vi "App - analyze RUS V6.vi"() -> ()   [LabVIEW 2018] (continued)
Data\\Ultrasound\\LSCO\\LSCO22__130814c\\5_Cooling_2nd_try\\September_2014\\091714\\54.81600K_500_2500_2.10000V_0.00000T_Sep17-2014__10-18-21_001_091714.bin", "mod time(min)"=58230138.35, "file format"=enum."binary", "power(V)"=2.1, "Magn Field(T) "=0.0}, {"temperature"=54.752, "temperature str"="54.75200", "file path"=path "D:/Data/Ultrasound/LSCO/LSCO22__130814c/5_Cooling_2nd_try/September_2014/091714/54.75200K_500_2500_2.10000V_0.00000T_Sep17-2014__10-19-41_001_091714.bin", "last mod"=timestamp(3493808381 s since 1904-01-01), "file name str"="D:\\Data\\Ultrasound\\LSCO\\LSCO22__130814c\\5_Cooling_2nd_try\\September_2014\\091714\\54.75200K_500_2500_2.10000V_0.00000T_Sep17-2014__10-19-41_001_091714.bin", "mod time(min)"=58230139.68333333, "file format"=enum."binary", "power(V)"=2.1, "Magn Field(T) "=0.0}, {"temperature"=54.691, "temperature str"="54.69100", "file path"=path "D:/Data/Ultrasound/LSCO/LSCO22__130814c/5_Cooling_2nd_try/September_2014/091714/54.69100K_500_2500_2.10000V_0.00000T_Sep17-2014__10-21-00_001_091714.bin", "last mod"=timestamp(3493808460 s since 1904-01-01), "file name str"="D:\\Data\\Ultrasound\\LSCO\\LSCO22__130814c\\5_Cooling_2nd_try\\September_2014\\091714\\54.69100K_500_2500_2.10000V_0.00000T_Sep17-2014__10-21-00_001_091714.bin", "mod time(min)"=58230141.0, "file format"=enum."binary", "power(V)"=2.1, "Magn Field(T) "=0.0}, {"temperature"=54.628, "temperature str"="54.62800", "file path"=path "D:/Data/Ultrasound/LSCO/LSCO22__130814c/5_Cooling_2nd_try/September_2014/091714/54.62800K_500_2500_2.10000V_0.00000T_Sep17-2014__10-22-19_001_091714.bin", "last mod"=timestamp(3493808539 s since 1904-01-01), "file name str"="D:\\Data\\Ultrasound\\LSCO\\LSCO22__130814c\\5_Cooling_2nd_try\\September_2014\\091714\\54.62800K_500_2500_2.10000V_0.00000T_Sep17-2014__10-22-19_001_091714.bin", "mod time(min)"=58230142.31666667, "file format"=enum."binary", "power(V)"=2.1, "Magn Field(T) "=0.0}, {"temperature"=54.564, "temperature str"="54.56400", "file path"=path "D:/Data/Ultrasound/LSCO/LSCO22__130814c/5_Cooling_2nd_try/September_2014/091714/54.56400K_500_2500_2.10000V_0.00000T_Sep17-2014__10-23-39_001_091714.bin", "last mod"=timestamp(3493808619 s since 1904-01-01), "file name str"="D:\\Data\\Ultrasound\\LSCO\\LSCO22__130814c\\5_Cooling_2nd_try\\September_2014\\091714\\54.56400K_500_2500_2.10000V_0.00000T_Sep17-2014__10-23-39_001_091714.bin", "mod time(min)"=58230143.65, "file format"=enum."binary", "power(V)"=2.1, "Magn Field(T) "=0.0}, {"temperature"=54.505, "temperature str"="54.50500", "file path"=path "D:/Data/Ultrasound/LSCO/LSCO22__130814c/5_Cooling_2nd_try/September_2014/091714/54.50500K_500_2500_2.10000V_0.00000T_Sep17-2014__10-24-58_001_091714.bin", "last mod"=timestamp(3493808698 s since 1904-01-01), "file name str"="D:\\Data\\Ultrasound\\LSCO\\LSCO22__130814c\\5_Cooling_2nd_try\\September_2014\\091714\\54.50500K_500_2500_2.10000V_0.00000T_Sep17-2014__10-24-58_001_091714.bin", "mod time(min)"=58230144.96666667, "file format"=enum."binary", "power(V)"=2.1, "Magn Field(T) "=0.0}, {"temperature"=54.44, "temperature str"="54.44000", "file path"=path "D:/Data/Ultrasound/LSCO/LSCO22__130814c/5_Cooling_2nd_try/September_2014/091714/54.44000K_500_2500_2.10000V_0.00000T_Sep17-2014__10-26-18_001_091714.bin", "last mod"=timestamp(3493808778 s since 1904-01-01), "file name str"="D:\\Data\\Ultrasound\\LSCO\\LSCO22__130814c\\5_Cooling_2nd_try\\September_2014\\091714\\54.44000K_500_2500_2.10000V_0.00000T_Sep17-2014__10-26-18_001_091714.bin", "mod time(min)"=58230146.3, "file format"=enum."binary", "power(V)"=2.1, "Magn Field(T) "=0.0}, {"temperature"=54.375, "temperature str"="54.37500", "file path"=path "D:/Data/Ultrasound/LSCO/LSCO22__130814c/5_Cooling_2nd_try/September_2014/091714/54.37500K_500_2500_2.10000V_0.00000T_Sep17-2014__10-27-37_001_091714.bin", "last mod"=timestamp(3493808857 s since 1904-01-01), "file name str"="D:\\Data\\Ultrasound\\LSCO\\LSCO22__130814c\\5_Cooling_2nd_try\\September_2014\\091714\\54.37500K_500_2500_2.10000V_0.00000T_Sep17-2014__10-27-37_001_091714.bin", "mod time(min)"=58230147.61666667, "file format"=enum."binary", "power(V)"=2.1, "Magn Field(T) "=0.0}, {"temperature"=54.316, "temperature str"="54.31600", "file path"=path "D:/Data/Ultrasound/LSCO/LSCO22__130814c/5_Cooling_2nd_try/September_2014/091714/54.31600K_500_2500_2.10000V_0.00000T_Sep17-2014__10-28-56_001_091714.bin", "last mod"=timestamp(3493808936 s since 1904-01-01), "file name str"="D:\\Data\\Ultrasound\\LSCO\\LSCO22__130814c\\5_Cooling_2nd_try\\September_2014\\091714\\54.31600K_500_2500_2.10000V_0.00000T_Sep17-2014__10-28-56_001_091714.bin", "mod time(min)"=58230148.93333333, "file format"=enum."binary", "power(V)"=2.1, "Magn Field(T) "=0.0}, {"temperature"=54.252, "temperature str"="54.25200", "file path"=path "D:/Data/Ultrasound/LSCO/LSCO22__130814c/5_Cooling_2nd_try/September_2014/091714/54.25200K_500_2500_2.10000V_0.00000T_Sep17-2014__10-30-16_001_091714.bin", "last mod"=timestamp(3493809016 s since 1904-01-01), "file name str"="D:\\Data\\Ultrasound\\LSCO\\LSCO22__130814c\\5_Cooling_2nd_try\\September_2014\\091714\\54.25200K_500_2500_2.10000V_0.00000T_Sep17-2014__10-30-16_001_091714.bin", "mod time(min)"=58230150.266666666, "file format"=enum."binary", "power(V)"=2.1, "Magn Field(T) "=0.0}, {"temperature"=54.191, "temperature str"="54.19100", "file path"=path "D:/Data/Ultrasound/LSCO/LSCO22__130814c/5_Cooling_2nd_try/September_2014/091714/54.19100K_500_2500_2.10000V_0.00000T_Sep17-2014__10-31-35_001_091714.bin", "last mod"=timestamp(3493809095 s since 1904-01-01), "file name str"="D:\\Data\\Ultrasound\\LSCO\\LSCO22__130814c\\5_Cooling_2nd_try\\September_2014\\091714\\54.19100K_500_2500_2.10000V_0.00000T_Sep17-2014__10-31-35_001_091714.bin", "mod time(min)"=58230151.583333336, "file format"=enum."binary", "power(V)"=2.1, "Magn Field(T) "=0.0}, {"temperature"=54.128, "temperature str"="54.12800", "file path"=path "D:/Data/Ultrasound/LSCO/LSCO22__130814c/5_Cooling_2nd_try/September_2014/091714/54.12800K_500_2500_2.10000V_0.00000T_Sep17-2014__10-32-54_001_091714.bin", "last mod"=timestamp(3493809174 s since 1904-01-01), "file name str"="D:\\Data\\Ultrasound\\LSCO\\LSCO22__130814c\\5_Cooling_2nd_try\\September_2014\\091714\\54.12800K_500_2500_2.10000V_0.00000T_Sep17-2014__10-32-54_001_091714.bin", "mod time(min)"=58230152.9, "file format"=enum."binary", "power(V)"=2.1, "Magn Field(T) "=0.0}, {"temperature"=54.064, "temperature str"="54.06400", "file path"=path "D:/Data/Ultrasound/LSCO/LSCO22__130814c/5_Cooling_2nd_try/September_2014/091714/54.06400K_500_2500_2.10000V_0.00000T_Sep17-2014__10-34-14_001_091714.bin", "last mod"=timestamp(3493809254 s since 1904-01-01), "file name str"="D:\\Data\\Ultrasound\\LSCO\\LSCO22__130814c\\5_Cooling_2nd_try\\September_2014\\091714\\54.06400K_500_2500_2.10000V_0.00000T_Sep17-2014__10-34-14_001_091714.bin", "mod time(min)"=58230154.233333334, "file format"=enum."binary", "power(V)"=2.1, "Magn Field(T) "=0.0}, {"temperature"=54.004, "temperature str"="54.00400", "file path"=path "D:/Data/Ultrasound/LSCO/LSCO22__130814c/5_Cooling_2nd_try/September_2014/091714/54.00400K_500_2500_2.10000V_0.00000T_Sep17-2014__10-35-33_001_091714.bin", "last mod"=timestamp(3493809333 s since 1904-01-01), "file name str"="D:\\Data\\Ultrasound\\LSCO\\LSCO22__130814c\\5_Cooling_2nd_try\\September_2014\\091714\\54.00400K_500_2500_2.10000V_0.00000T_Sep17-2014__10-35-33_001_091714.bin", "mod time(min)"=58230155.55, "file format"=enum."binary", "power(V)"=2.1, "Magn Field(T) "=0.0}, {"temperature"=53.936, "temperature str"="53.93600", "file path"=path "D:/Data/Ultrasound/LSCO/LSCO22__130814c/5_Cooling_2nd_try/September_2014/091714/53.93600K_500_2500_2.10000V_0.00000T_Sep17-2014__10-36-53_001_091714.bin", "last mod"=timestamp(3493809413 s since 1904-01-01), "file name str"="D:\\Data\\Ultrasound\\LSCO\\LSCO22__130814c\\5_Cooling_2nd_try\\September_2014\\091714\\53.93600K_500_2500_2.10000V_0.00000T_Sep17-2014__10-36-53_001_091714.bin", "mod time(min)"=58230156.88333333, "file format"=enum."binary", "power(V)"=2.1, "Magn Field(T) "=0.0}, {"temperature"=53.874, "temperature str"="53.87400", "file path"=path "D:/Data/Ultrasound/LSCO/LSCO22__130814c/5_Cooling_2nd_try/September_2014/091714/53.87400K_500_2500_2.10000V_0.00000T_Sep17-2014__10-38-12_001_091714.bin", "last mod"=timestamp(3493809492 s since 1904-01-01), "file name str"="D:\\Data\\Ultrasound\\LSCO\\LSCO22__130814c\\5_Cooling_2nd_try\\September_2014\\091714\\53.87400K_500_2500_2.10000V_0.00000T_Sep17-2014__10-38-12_001_091714.bin", "mod time(min)"=58230158.2, "file format"=enum."binary", "power(V)"=2.1, "Magn Field(T) "=0.0}, {"temperature"=53.813, "temperature str"="53.81300", "file path"=path "D:/Data/Ultrasound/LSCO/LSCO22__130814c/5_Cooling_2nd_try/September_2014/091714/53.81300K_500_2500_2.10000V_0.00000T_Sep17-2014__10-39-31_001_091714.bin", "last mod"=timestamp(3493809571 s since 1904-01-01), "file name str"="D:\\Data\\Ultrasound\\LSCO\\LSCO22__130814c\\5_Cooling_2nd_try\\September_2014\\091714\\53.81300K_500_2500_2.10000V_0.00000T_Sep17-2014__10-39-31_001_091714.bin", "mod time(min)"=58230159.516666666, "file format"=enum."binary", "power(V)"=2.1, "Magn Field(T) "=0.0}, {"temperature"=53.746, "temperature str"="53.74600", "file path"=path "D:/Data/Ultrasound/LSCO/LSCO22__130814c/5_Cooling_2nd_try/September_2014/091714/53.74600K_500_2500_2.10000V_0.00000T_Sep17-2014__10-40-51_001_091714.bin", "last mod"=timestamp(3493809651 s since 1904-01-01), "file name str"="D:\\Data\\Ultrasound\\LSCO\\LSCO22__130814c\\5_Cooling_2nd_try\\September_2014\\091714\\53.74600K_500_2500_2.10000V_0.00000T_Sep17-2014__10-40-51_001_091714.bin", "mod time(min)"=58230160.85, "file format"=enum."binary", "power(V)"=2.1, "Magn Field(T) "=0.0}, {"temperature"=53.683, "temperature str"="53.68300", "file path"=path "D:/Data/Ultrasound/LSCO/LSCO22__130814c/5_Cooling_2nd_try/September_2014/091714/53.68300K_500_2500_2.10000V_0.00000T_Sep17-2014__10-42-10_001_091714.bin", "last mod"=timestamp(3493809730 s since 1904-01-01), "file name str"="D:\\Data\\Ultrasound\\LSCO\\LSCO22__130814c\\5_Cooling_2nd_try\\September_2014\\091714\\53.68300K_500_2500_2.10000V_0.00000T_Sep17-2014__10-42-10_001_091714.bin", "mod time(min)"=58230162.166666664, "file format"=enum."binary", "power(V)"=2.1, "Magn Field(T) "=0.0}, {"temperature"=53.622, "temperature str"="53.62200", "file path"=path "D:/Data/Ultrasound/LSCO/LSCO22__130814c/5_Cooling_2nd_try/September_2014/091714/53.62200K_500_2500_2.10000V_0.00000T_Sep17-2014__10-43-29_001_091714.bin", "last mod"=timestamp(3493809809 s since 1904-01-01), "file name str"="D:\\Data\\Ultrasound\\LSCO\\LSCO22__130814c\\5_Cooling_2nd_try\\September_2014\\091714\\53.62200K_500_2500_2.10000V_0.00000T_Sep17-2014__10-43-29_001_091714.bin", "mod time(min)"=58230163.483333334, "file format"=enum."binary", "power(V)"=2.1, "Magn Field(T) "=0.0}, {"temperature"=53.557, "temperature str"="53.55700", "file path"=path "D:/Data/Ultrasound/LSCO/LSCO22__130814c/5_Cooling_2nd_try/September_2014/091714/53.55700K_500_2500_2.10000V_0.00000T_Sep17-2014__10-44-49_001_091714.bin", "last mod"=timestamp(3493809889 s since 1904-01-01), "file name str"="D:\\Data\\Ultrasound\\LSCO\\LSCO22__130814c\\5_Cooling_2nd_try\\September_2014\\091714\\53.55700K_500_2500_2.10000V_0.00000T_Sep17-2014__10-44-49_001_091714.bin", "mod time(min)"=58230164.81666667, "file format"=enum."binary", "power(V)"=2.1, "Magn Field(T) "=0.0}, {"temperature"=53.492, "temperature str"="53.49200", "file path"=path "D:/Data/Ultrasound/LSCO/LSCO22__130814c/5_Cooling_2nd_try/September_2014/091714/53.49200K_500_2500_2.10000V_0.00000T_Sep17-2014__10-46-08_001_091714.bin", "last mod"=timestamp(3493809968 s since 1904-01-01), "file name str"="D:\\Data\\Ultrasound\\LSCO\\LSCO22__130814c\\5_Cooling_2nd_try\\September_2014\\091714\\53.49200K_500_2500_2.10000V_0.00000T_Sep17-2014__10-46-08_001_091714.bin", "mod time(min)"=58230166.13333333, "file format"=enum."binary", "power(V)"=2.1, "Magn Field(T) "=0.0}, {"temperature"=53.431, "temperature str"="53.43100", "file path"=path "D:/Data/Ultrasound/LSCO/LSCO22__130814c/5_Cooling_2nd_try/September_2014/091714/53.43100K_500_2500_2.10000V_0.00000T_Sep17-2014__10-47-28_001_091714.bin", "last mod"=timestamp(3493810048 s since 1904-01-01), "file name str"="D:\\Data\\Ultrasound\\LSCO\\LSCO22__130814c\\5_Cooling_2nd_try\\September_2014\\091714\\53.43100K_500_2500_2.10000V_0.00000T_Sep17-2014__10-47-28_001_091714.bin", "mod time(min)"=58230167.46666667, "file format"=enum."binary", "power(V)"=2.1, "Magn Field(T) "=0.0}, {"temperature"=53.368, "temperature str"="53.36800", "file path"=path "D:/Data/Ultrasound/LSCO/LSCO22__130814c/5_Cooling_2nd_try/September_2014/091714/53.36800K_500_2500_2.10000V_0.00000T_Sep17-2014__10-48-47_001_091714.bin", "last mod"=timestamp(3493810127 s since 1904-01-01), "file name str"="D:\\Data\\Ultrasound\\LSCO\\LSCO22__130814c\\5_Cooling_2nd_try\\September_2014\\091714\\53.36800K_500_2500_2.10000V_0.00000T_Sep17-2014__10-48-47_001_091714.bin", "mod time(min)"=58230168.78333333, "file format"=enum."binary", "power(V)"=2.1, "Magn Field(T) "=0.0}, {"temperature"=53.304, "temperature str"="53.30400", "file path"=path "D:/Data/Ultrasound/LSCO/LSCO22__130814c/5_Cooling_2nd_try/September_2014/091714/53.30400K_500_2500_2.10000V_0.00000T_Sep17-2014__10-50-06_001_091714.bin", "last mod"=timestamp(3493810206 s since 1904-01-01), "file name str"="D:\\Data\\Ultrasound\\LSCO\\LSCO22__130814c\\5_Cooling_2nd_try\\September_2014\\091714\\53.30400K_500_2500_2.10000V_0.00000T_Sep17-2014__10-50-06_001_091714.bin", "mod time(min)"=58230170.1, "file format"=enum."binary", "power(V)"=2.1, "Magn Field(T) "=0.0}, {"temperature"=53.234, "temperature str"="53.23400", "file path"=path "D:/Data/Ultrasound/LSCO/LSCO22__130814c/5_Cooling_2nd_try/September_2014/091714/53.23400K_500_2500_2.10000V_0.00000T_Sep17-2014__10-51-26_001_091714.bin", "last mod"=timestamp(3493810286 s since 1904-01-01), "file name str"="D:\\Data\\Ultrasound\\LSCO\\LSCO22__130814c\\5_Cooling_2nd_try\\September_2014\\091714\\53.23400K_500_2500_2.10000V_0.00000T_Sep17-2014__10-51-26_001_091714.bin", "mod time(min)"=58230171.43333333, "file format"=enum."binary", "power(V)"=2.1, "Magn Field(T) "=0.0}, {"temperature"=53.178, "temperature str"="53.17800", "file path"=path "D:/Data/Ultrasound/LSCO/LSCO22__130814c/5_Cooling_2nd_try/September_2014/091714/53.17800K_500_2500_2.10000V_0.00000T_Sep17-2014__10-52-45_001_091714.bin", "last mod"=timestamp(3493810365 s since 1904-01-01), "file name str"="D:\\Data\\Ultrasound\\LSCO\\LSCO22__130814c\\5_Cooling_2nd_try\\September_2014\\091714\\53.17800K_500_2500_2.10000V_0.00000T_Sep17-2014__10-52-45_001_091714.bin", "mod time(min)"=58230172.75, "file format"=enum."binary", "power(V)"=2.1, "Magn Field(T) "=0.0}, {"temperature"=53.112, "temperature str"="53.11200", "file path"=path "D:/Data/Ultrasound/LSCO/LSCO22__130814c/5_Cooling_2nd_try/September_2014/091714/53.11200K_500_2500_2.10000V_0.00000T_Sep17-2014__10-54-04_001_091714.bin", "last mod"=timestamp(3493810444 s since 1904-01-01), "file name str"="D:\\Data\\Ultrasound\\LSCO\\LSCO22__130814c\\5_Cooling_2nd_try\\September_2014\\091714\\53.11200K_500_2500_2.10000V_0.00000T_Sep17-2014__10-54-04_001_091714.bin", "mod time(min)"=58230174.06666667, "file format"=enum."binary", "power(V)"=2.1, "Magn Field(T) "=0.0}, {"temperature"=53.046, "temperature str"="53.04600", "file path"=path "D:/Data/Ultrasound/LSCO/LSCO22__130814c/5_Cooling_2nd_try/September_2014/091714/53.04600K_500_2500_2.10000V_0.00000T_Sep17-2014__10-55-24_001_091714.bin", "last mod"=timestamp(3493810524 s since 1904-01-01), "file name str"="D:\\Data\\Ultrasound\\LSCO\\LSCO22__130814c\\5_Cooling_2nd_try\\September_2014\\091714\\53.04600K_500_2500_2.10000V_0.00000T_Sep17-2014__10-55-24_001_091714.bin", "mod time(min)"=58230175.4, "file format"=enum."binary", "power(V)"=2.1, "Magn Field(T) "=0.0}, {"temperature"=52.981, "temperature str"="52.98100", "file path"=path "D:/Data/Ultrasound/LSCO/LSCO22__130814c/5_Cooling_2nd_try/September_2014/091714/52.98100K_500_2500_2.10000V_0.00000T_Sep17-2014__10-56-43_001_091714.bin", "last mod"=timestamp(3493810603 s since 1904-01-01), "file name str"="D:\\Data\\Ultrasound\\LSCO\\LSCO22__130814c\\5_Cooling_2nd_try\\September_2014\\091714\\52.98100K_500_2500_2.10000V_0.00000T_Sep17-2014__10-56-43_001_091714.bin", "mod time(min)"=58230176.71666667, "file format"=enum."binary", "power(V)"=2.1, "Magn Field(T) "=0.0}, {"temperature"=52.922, "temperature str"="52.92200", "file path"=path "D:/Data/Ultrasound/LSCO/LSCO22__130814c/5_Cooling_2nd_try/September_2014/091714/52.92200K_500_2500_2.10000V_0.00000T_Sep17-2014__10-58-03_001_091714.bin", "last mod"=timestamp(3493810683 s since 1904-01-01), "file name str"="D:\\Data\\Ultrasound\\LSCO\\LSCO22__130814c\\5_Cooling_2nd_try\\September_2014\\091714\\52.92200K_500_2500_2.10000V_0.00000T_Sep17-2014__10-58-03_001_091714.bin", "mod time(min)"=58230178.05, "file format"=enum."binary", "power(V)"=2.1, "Magn Field(T) "=0.0}, {"temperature"=52.856, "temperature str"="52.85600", "file path"=path "D:/Data/Ultrasound/LSCO/LSCO22__130814c/5_Cooling_2nd_try/September_2014/091714/52.85600K_500_2500_2.10000V_0.00000T_Sep17-2014__10-59-22_001_091714.bin", "last mod"=timestamp(3493810762 s since 1904-01-01), "file name str"="D:\\Data\\Ultrasound\\LSCO\\LSCO22__130814c\\5_Cooling_2nd_try\\September_2014\\091714\\52.85600K_500_2500_2.10000V_0.00000T_Sep17-2014__10-59-22_001_091714.bin", "mod time(min)"=58230179.36666667, "file format"=enum."binary", "power(V)"=2.1, "Magn Field(T) "=0.0}, {"temperature"=52.786, "temperature str"="52.78600", "file path"=path "D:/Data/Ultrasound/LSCO/LSCO22__130814c/5_Cooling_2nd_try/September_2014/091714/52.78600K_500_2500_2.10000V_0.00000T_Sep17-2014__11-00-41_001_091714.bin", "last mod"=timestamp(3493810841 s since 1904-01-01), "file name str"="D:\\Data\\Ultrasound\\LSCO\\LSCO22__130814c\\5_Cooling_2nd_try\\September_2014\\091714\\52.78600K_500_2500_2.10000V_0.00000T_Sep17-2014__11-00-41_001_091714.bin", "mod time(min)"=58230180.68333333, "file format"=enum."binary", "power(V)"=2.1, "Magn Field(T) "=0.0}, {"temperature"=52.726, "temperature str"="52.72600", "file path"=path "D:/Data/Ultrasound/LSCO/LSCO22__130814c/5_Cooling_2nd_try/September_2014/091714/52.72600K_500_2500_2.10000V_0.00000T_Sep17-2014__11-02-01_001_091714.bin", "last mod"=timestamp(3493810921 s since 1904-01-01), "file name str"="D:\\Data\\Ultrasound\\LSCO\\LSCO22__130814c\\5_Cooling_2nd_try\\September_2014\\091714\\52.72600K_500_2500_2.10000V_0.00000T_Sep17-2014__11-02-01_001_091714.bin", "mod time(min)"=58230182.016666666, "file format"=enum."binary", "power(V)"=2.1, "Magn Field(T) "=0.0}, {"temperature"=52.665, "temperature str"="52.66500", "file path"=path "D:/Data/Ultrasound/LSCO/LSCO22__130814c/5_Cooling_2nd_try/September_2014/091714/52.66500K_500_2500_2.10000V_0.00000T_Sep17-2014__11-03-20_001_091714.bin", "last mod"=timestamp(3493811000 s since 1904-01-01), "file name str"="D:\\Data\\Ultrasound\\LSCO\\LSCO22__130814c\\5_Cooling_2nd_try\\September_2014\\091714\\52.66500K_500_2500_2.10000V_0.00000T_Sep17-2014__11-03-20_001_091714.bin", "mod time(min)"=58230183.333333336, "file format"=enum."binary", "power(V)"=2.1, "Magn Field(T) "=0.0}, {"temperature"=52.593, "temperature str"="52.59300", "file path"=path "D:/Data/Ultrasound/LSCO/LSCO22__130814c/5_Cooling_2nd_try/September_2014/091714/52.59300K_500_2500_2.10000V_0.00000T_Sep17-2014__11-04-39_001_091714.bin", "last mod"=timestamp(3493811079 s since 1904-01-01), "file name str"="D:\\Data\\Ultrasound\\LSCO\\LSCO22__130814c\\5_Cooling_2nd_try\\September_2014\\091714\\52.59300K_500_2500_2.10000V_0.00000T_Sep17-2014__11-04-39_001_091714.bin", "mod time(min)"=58230184.65, "file format"=enum."binary", "power(V)"=2.1, "Magn Field(T) "=0.0}, {"temperature"=52.53, "temperature str"="52.53000", "file path"=path "D:/Data/Ultrasound/LSCO/LSCO22__130814c/5_Cooling_2nd_try/September_2014/091714/52.53000K_500_2500_2.10000V_0.00000T_Sep17-2014__11-05-59_001_091714.bin", "last mod"=timestamp(3493811159 s since 1904-01-01), "file name str"="D:\\Data\\Ultrasound\\LSCO\\LSCO22__130814c\\5_Cooling_2nd_try\\September_2014\\091714\\52.53000K_500_2500_2.10000V_0.00000T_Sep17-2014__11-05-59_001_091714.bin", "mod time(min)"=58230185.983333334, "file format"=enum."binary", "power(V)"=2.1, "Magn Field(T) "=0.0}, {"temperature"=52.467, "temperature str"="52.46700", "file path"=path "D:/Data/Ultrasound/LSCO/LSCO22__130814c/5_Cooling_2nd_try/September_2014/091714/52.46700K_500_2500_2.10000V_0.00000T_Sep17-2014__11-07-18_001_091714.bin", "last mod"=timestamp(3493811238 s since 1904-01-01), "file name str"="D:\\Data\\Ultrasound\\LSCO\\LSCO22__130814c\\5_Cooling_2nd_try\\September_2014\\091714\\52.46700K_500_2500_2.10000V_0.00000T_Sep17-2014__11-07-18_001_091714.bin", "mod time(min)"=58230187.3, "file format"=enum."binary", "power(V)"=2.1, "Magn Field(T) "=0.0}, {"temperature"=52.405, "temperature str"="52.40500", "file path"=path "D:/Data/Ultrasound/LSCO/LSCO22__130814c/5_Cooling_2nd_try/September_2014/091714/52.40500K_500_2500_2.10000V_0.00000T_Sep17-2014__11-08-38_001_091714.bin", "last mod"=timestamp(3493811318 s since 1904-01-01), "file name str"="D:\\Data\\Ultrasound\\LSCO\\LSCO22__130814c\\5_Cooling_2nd_try\\September_2014\\091714\\52.40500K_500_2500_2.10000V_0.00000T_Sep17-2014__11-08-38_001_091714.bin", "mod time(min)"=58230188.63333333, "file format"=enum."binary", "power(V)"=2.1, "Magn Field(T) "=0.0}, {"temperature"=52.337, "temperature str"="52.33700", "file path"=path "D:/Data/Ultrasound/LSCO/LSCO22__130814c/5_Cooling_2nd_try/September_2014/091714/52.33700K_500_2500_2.10000V_0.00000T_Sep17-2014__11-09-57_001_091714.bin", "last mod"=timestamp(3493811397 s since 1904-01-01), "file name str"="D:\\Data\\Ultrasound\\LSCO\\LSCO22__130814c\\5_Cooling_2nd_try\\September_2014\\091714\\52.33700K_500_2500_2.10000V_0.00000T_Sep17-2014__11-09-57_001_091714.bin", "mod time(min)"=58230189.95, "file format"=enum."binary", "power(V)"=2.1, "Magn Field(T) "=0.0}, {"temperature"=52.27, "temperature str"="52.27000", "file path"=path "D:/Data/Ultrasound/LSCO/LSCO22__130814c/5_Cooling_2nd_try/September_2014/091714/52.27000K_500_2500_2.10000V_0.00000T_Sep17-2014__11-11-16_001_091714.bin", "last mod"=timestamp(3493811476 s since 1904-01-01), "file name str"="D:\\Data\\Ultrasound\\LSCO\\LSCO22__130814c\\5_Cooling_2nd_try\\September_2014\\091714\\52.27000K_500_2500_2.10000V_0.00000T_Sep17-2014__11-11-16_001_091714.bin", "mod time(min)"=58230191.266666666, "file format"=enum."binary", "power(V)"=2.1, "Magn Field(T) "=0.0}, {"temperature"=52.209, "temperature str"="52.20900", "file path"=path "D:/Data/Ultrasound/LSCO/LSCO22__130814c/5_Cooling_2nd_try/September_2014/091714/52.20900K_500_2500_2.10000V_0.00000T_Sep17-2014__11-12-36_001_091714.bin", "last mod"=timestamp(3493811556 s since 1904-01-01), "file name str"="D:\\Data\\Ultrasound\\LSCO\\LSCO22__130814c\\5_Cooling_2nd_try\\September_2014\\091714\\52.20900K_500_2500_2.10000V_0.00000T_Sep17-2014__11-12-36_001_091714.bin", "mod time(min)"=58230192.6, "file format"=enum."binary", "power(V)"=2.1, "Magn Field(T) "=0.0}, {"temperature"=52.142, "temperature str"="52.14200", "file path"=path "D:/Data/Ultrasound/LSCO/LSCO22__130814c/5_Cooling_2nd_try/September_2014/091714/52.14200K_500_2500_2.10000V_0.00000T_Sep17-2014__11-13-55_001_091714.bin", "last mod"=timestamp(3493811635 s since 1904-01-01), "file name str"="D:\\Data\\Ultrasound\\LSCO\\LSCO22__130814c\\5_Cooling_2nd_try\\September_2014\\091714\\52.14200K_500_2500_2.10000V_0.00000T_Sep17-2014__11-13-55_001_091714.bin", "mod time(min)"=58230193.916666664, "file format"=enum."binary", "power(V)"=2.1, "Magn Field(T) "=0.0}, {"temperature"=52.081, "temperature str"="52.08100", "file path"=path "D:/Data/Ultrasound/LSCO/LSCO22__130814c/5_Cooling_2nd_try/September_2014/091714/52.08100K_500_2500_2.10000V_0.00000T_Sep17-2014__11-15-14_001_091714.bin", "last mod"=timestamp(3493811714 s since 1904-01-01), "file name str"="D:\\Data\\Ultrasound\\LSCO\\LSCO22__130814c\\5_Cooling_2nd_try\\September_2014\\091714\\52.08100K_500_2500_2.10000V_0.00000T_Sep17-2014__11-15-14_001_091714.bin", "mod time(min)"=58230195.233333334, "file format"=enum."binary", "power(V)"=2.1, "Magn Field(T) "=0.0}, {"temperature"=52.015, "temperature str"="52.01500", "file path"=path "D:/Data/Ultrasound/LSCO/LSCO22__130814c/5_Cooling_2nd_try/September_2014/091714/52.01500K_500_2500_2.10000V_0.00000T_Sep17-2014__11-16-34_001_091714.bin", "last mod"=timestamp(3493811794 s since 1904-01-01), "file name str"="D:\\Data\\Ultrasound\\LSCO\\LSCO22__130814c\\5_Cooling_2nd_try\\September_2014\\091714\\52.01500K_500_2500_2.10000V_0.00000T_Sep17-2014__11-16-34_001_091714.bin", "mod time(min)"=58230196.56666667, "file format"=enum."binary", "power(V)"=2.1, "Magn Field(T) "=0.0}, {"temperature"=51.945, "temperature str"="51.94500", "file path"=path "D:/Data/Ultrasound/LSCO/LSCO22__130814c/5_Cooling_2nd_try/September_2014/091714/51.94500K_500_2500_2.10000V_0.00000T_Sep17-2014__11-17-53_001_091714.bin", "last mod"=timestamp(3493811873 s since 1904-01-01), "file name str"="D:\\Data\\Ultrasound\\LSCO\\LSCO22__130814c\\5_Cooling_2nd_try\\September_2014\\091714\\51.94500K_500_2500_2.10000V_0.00000T_Sep17-2014__11-17-53_001_091714.bin", "mod time(min)"=58230197.88333333, "file format"=enum."binary", "power(V)"=2.1, "Magn Field(T) "=0.0}, {"temperature"=51.883, "temperature str"="51.88300", "file path"=path "D:/Data/Ultrasound/LSCO/LSCO22__130814c/5_Cooling_2nd_try/September_2014/091714/51.88300K_500_2500_2.10000V_0.00000T_Sep17-2014__11-19-12_001_091714.bin", "last mod"=timestamp(3493811952 s since 1904-01-01), "file name str"="D:\\Data\\Ultrasound\\LSCO\\LSCO22__130814c\\5_Cooling_2nd_try\\September_2014\\091714\\51.88300K_500_2500_2.10000V_0.00000T_Sep17-2014__11-19-12_001_091714.bin", "mod time(min)"=58230199.2, "file format"=enum."binary", "power(V)"=2.1, "Magn Field(T) "=0.0}, {"temperature"=51.82, "temperature str"="51.82000", "file path"=path "D:/Data/Ultrasound/LSCO/LSCO22__130814c/5_Cooling_2nd_try/September_2014/091714/51.82000K_500_2500_2.10000V_0.00000T_Sep17-2014__11-20-32_001_091714.bin", "last mod"=timestamp(3493812032 s since 1904-01-01), "file name str"="D:\\Data\\Ultrasound\\LSCO\\LSCO22__130814c\\5_Cooling_2nd_try\\September_2014\\091714\\51.82000K_500_2500_2.10000V_0.00000T_Sep17-2014__11-20-32_001_091714.bin", "mod time(min)"=58230200.53333333, "file format"=enum."binary", "power(V)"=2.1, "Magn Field(T) "=0.0}, {"temperature"=51.755, "temperature str"="51.75500", "file path"=path "D:/Data/Ultrasound/LSCO/LSCO22__130814c/5_Cooling_2nd_try/September_2014/091714/51.75500K_500_2500_2.10000V_0.00000T_Sep17-2014__11-21-51_001_091714.bin", "last mod"=timestamp(3493812111 s since 1904-01-01), "file name str"="D:\\Data\\Ultrasound\\LSCO\\LSCO22__130814c\\5_Cooling_2nd_try\\September_2014\\091714\\51.75500K_500_2500_2.10000V_0.00000T_Sep17-2014__11-21-51_001_091714.bin", "mod time(min)"=58230201.85, "file format"=enum."binary", "power(V)"=2.1, "Magn Field(T) "=0.0}, {"temperature"=51.682, "temperature str"="51.68200", "file path"=path "D:/Data/Ultrasound/LSCO/LSCO22__130814c/5_Cooling_2nd_try/September_2014/091714/51.68200K_500_2500_2.10000V_0.00000T_Sep17-2014__11-23-11_001_091714.bin", "last mod"=timestamp(3493812191 s since 1904-01-01), "file name str"="D:\\Data\\Ultrasound\\LSCO\\LSCO22__130814c\\5_Cooling_2nd_try\\September_2014\\091714\\51.68200K_500_2500_2.10000V_0.00000T_Sep17-2014__11-23-11_001_091714.bin", "mod time(min)"=58230203.18333333, "file format"=enum."binary", "power(V)"=2.1, "Magn Field(T) "=0.0}, {"temperature"=51.621, "temperature str"="51.62100", "file path"=path "D:/Data/Ultrasound/LSCO/LSCO22__130814c/5_Cooling_2nd_try/September_2014/091714/51.62100K_500_2500_2.10000V_0.00000T_Sep17-2014__11-24-30_001_091714.bin", "last mod"=timestamp(3493812270 s since 1904-01-01), "file name str"="D:\\Data\\Ultrasound\\LSCO\\LSCO22__130814c\\5_Cooling_2nd_try\\September_2014\\091714\\51.62100K_500_2500_2.10000V_0.00000T_Sep17-2014__11-24-30_001_091714.bin", "mod time(min)"=58230204.5, "file format"=enum."binary", "power(V)"=2.1, "Magn Field(T) "=0.0}, {"temperature"=51.556, "temperature str"="51.55600", "file path"=path "D:/Data/Ultrasound/LSCO/LSCO22__130814c/5_Cooling_2nd_try/September_2014/091714/51.55600K_500_2500_2.10000V_0.00000T_Sep17-2014__11-25-49_001_091714.bin", "last mod"=timestamp(3493812349 s since 1904-01-01), "file name str"="D:\\Data\\Ultrasound\\LSCO\\LSCO22__130814c\\5_Cooling_2nd_try\\September_2014\\091714\\51.55600K_500_2500_2.10000V_0.00000T_Sep17-2014__11-25-49_001_091714.bin", "mod time(min)"=58230205.81666667, "file format"=enum."binary", "power(V)"=2.1, "Magn Field(T) "=0.0}, {"temperature"=51.489, "temperature str"="51.48900", "file path"=path "D:/Data/Ultrasound/LSCO/LSCO22__130814c/5_Cooling_2nd_try/September_2014/091714/51.48900K_500_2500_2.10000V_0.00000T_Sep17-2014__11-27-09_001_091714.bin", "last mod"=timestamp(3493812429 s since 1904-01-01), "file name str"="D:\\Data\\Ultrasound\\LSCO\\LSCO22__130814c\\5_Cooling_2nd_try\\September_2014\\091714\\51.48900K_500_2500_2.10000V_0.00000T_Sep17-2014__11-27-09_001_091714.bin", "mod time(min)"=58230207.15, "file format"=enum."binary", "power(V)"=2.1, "Magn Field(T) "=0.0}, {"temperature"=51.422, "temperature str"="51.42200", "file path"=path "D:/Data/Ultrasound/LSCO/LSCO22__130814c/5_Cooling_2nd_try/September_2014/091714/51.42200K_500_2500_2.10000V_0.00000T_Sep17-2014__11-28-28_001_091714.bin", "last mod"=timestamp(3493812508 s since 1904-01-01), "file name str"="D:\\Data\\Ultrasound\\LSCO\\LSCO22__130814c\\5_Cooling_2nd_try\\September_2014\\091714\\51.42200K_500_2500_2.10000V_0.00000T_Sep17-2014__11-28-28_001_091714.bin", "mod time(min)"=58230208.46666667, "file format"=enum."binary", "power(V)"=2.1, "Magn Field(T) "=0.0}, {"temperature"=51.358, "temperature str"="51.35800", "file path"=path "D:/Data/Ultrasound/LSCO/LSCO22__130814c/5_Cooling_2nd_try/September_2014/091714/51.35800K_500_2500_2.10000V_0.00000T_Sep17-2014__11-29-47_001_091714.bin", "last mod"=timestamp(3493812587 s since 1904-01-01), "file name str"="D:\\Data\\Ultrasound\\LSCO\\LSCO22__130814c\\5_Cooling_2nd_try\\September_2014\\091714\\51.35800K_500_2500_2.10000V_0.00000T_Sep17-2014__11-29-47_001_091714.bin", "mod time(min)"=58230209.78333333, "file format"=enum."binary", "power(V)"=2.1, "Magn Field(T) "=0.0}, {"temperature"=51.292, "temperature str"="51.29200", "file path"=path "D:/Data/Ultrasound/LSCO/LSCO22__130814c/5_Cooling_2nd_try/September_2014/091714/51.29200K_500_2500_2.10000V_0.00000T_Sep17-2014__11-31-07_001_091714.bin", "last mod"=timestamp(3493812667 s since 1904-01-01), "file name str"="D:\\Data\\Ultrasound\\LSCO\\LSCO22__130814c\\5_Cooling_2nd_try\\September_2014\\091714\\51.29200K_500_2500_2.10000V_0.00000T_Sep17-2014__11-31-07_001_091714.bin", "mod time(min)"=58230211.11666667, "file format"=enum."binary", "power(V)"=2.1, "Magn Field(T) "=0.0}, {"temperature"=51.226, "temperature str"="51.22600", "file path"=path "D:/Data/Ultrasound/LSCO/LSCO22__130814c/5_Cooling_2nd_try/September_2014/091714/51.22600K_500_2500_2.10000V_0.00000T_Sep17-2014__11-32-26_001_091714.bin", "last mod"=timestamp(3493812746 s since 1904-01-01), "file name str"="D:\\Data\\Ultrasound\\LSCO\\LSCO22__130814c\\5_Cooling_2nd_try\\September_2014\\091714\\51.22600K_500_2500_2.10000V_0.00000T_Sep17-2014__11-32-26_001_091714.bin", "mod time(min)"=58230212.43333333, "file format"=enum."binary", "power(V)"=2.1, "Magn Field(T) "=0.0}, {"temperature"=51.159, "temperature str"="51.15900", "file path"=path "D:/Data/Ultrasound/LSCO/LSCO22__130814c/5_Cooling_2nd_try/September_2014/091714/51.15900K_500_2500_2.10000V_0.00000T_Sep17-2014__11-33-46_001_091714.bin", "last mod"=timestamp(3493812826 s since 1904-01-01), "file name str"="D:\\Data\\Ultrasound\\LSCO\\LSCO22__130814c\\5_Cooling_2nd_try\\September_2014\\091714\\51.15900K_500_2500_2.10000V_0.00000T_Sep17-2014__11-33-46_001_091714.bin", "mod time(min)"=58230213.766666666, "file format"=enum."binary", "power(V)"=2.1, "Magn Field(T) "=0.0}, {"temperature"=51.091, "temperature str"="51.09100", "file path"=path "D:/Data/Ultrasound/LSCO/LSCO22__130814c/5_Cooling_2nd_try/September_2014/091714/51.09100K_500_2500_2.10000V_0.00000T_Sep17-2014__11-35-05_001_091714.bin", "last mod"=timestamp(3493812905 s since 1904-01-01), "file name str"="D:\\Data\\Ultrasound\\LSCO\\LSCO22__130814c\\5_Cooling_2nd_try\\September_2014\\091714\\51.09100K_500_2500_2.10000V_0.00000T_Sep17-2014__11-35-05_001_091714.bin", "mod time(min)"=58230215.083333336, "file format"=enum."binary", "power(V)"=2.1, "Magn Field(T) "=0.0}, {"temperature"=51.03, "temperature str"="51.03000", "file path"=path "D:/Data/Ultrasound/LSCO/LSCO22__130814c/5_Cooling_2nd_try/September_2014/091714/51.03000K_500_2500_2.10000V_0.00000T_Sep17-2014__11-36-24_001_091714.bin", "last mod"=timestamp(3493812984 s since 1904-01-01), "file name str"="D:\\Data\\Ultrasound\\LSCO\\LSCO22__130814c\\5_Cooling_2nd_try\\September_2014\\091714\\51.03000K_500_2500_2.10000V_0.00000T_Sep17-2014__11-36-24_001_091714.bin", "mod time(min)"=58230216.4, "file format"=enum."binary", "power(V)"=2.1, "Magn Field(T) "=0.0}, {"temperature"=50.958, "temperature str"="50.95800", "file path"=path "D:/Data/Ultrasound/LSCO/LSCO22__130814c/5_Cooling_2nd_try/September_2014/091714/50.95800K_500_2500_2.10000V_0.00000T_Sep17-2014__11-37-44_001_091714.bin", "last mod"=timestamp(3493813064 s since 1904-01-01), "file name str"="D:\\Data\\Ultrasound\\LSCO\\LSCO22__130814c\\5_Cooling_2nd_try\\September_2014\\091714\\50.95800K_500_2500_2.10000V_0.00000T_Sep17-2014__11-37-44_001_091714.bin", "mod time(min)"=58230217.733333334, "file format"=enum."binary", "power(V)"=2.1, "Magn Field(T) "=0.0}, {"temperature"=50.9, "temperature str"="50.90000", "file path"=path "D:/Data/Ultrasound/LSCO/LSCO22__130814c/5_Cooling_2nd_try/September_2014/091714/50.90000K_500_2500_2.10000V_0.00000T_Sep17-2014__11-39-03_001_091714.bin", "last mod"=timestamp(3493813143 s since 1904-01-01), "file name str"="D:\\Data\\Ultrasound\\LSCO\\LSCO22__130814c\\5_Cooling_2nd_try\\September_2014\\091714\\50.90000K_500_2500_2.10000V_0.00000T_Sep17-2014__11-39-03_001_091714.bin", "mod time(min)"=58230219.05, "file format"=enum."binary", "power(V)"=2.1, "Magn Field(T) "=0.0}, {"temperature"=50.832, "temperature str"="50.83200", "file path"=path "D:/Data/Ultrasound/LSCO/LSCO22__130814c/5_Cooling_2nd_try/September_2014/091714/50.83200K_500_2500_2.10000V_0.00000T_Sep17-2014__11-40-23_001_091714.bin", "last mod"=timestamp(3493813223 s since 1904-01-01), "file name str"="D:\\Data\\Ultrasound\\LSCO\\LSCO22__130814c\\5_Cooling_2nd_try\\September_2014\\091714\\50.83200K_500_2500_2.10000V_0.00000T_Sep17-2014__11-40-23_001_091714.bin", "mod time(min)"=58230220.38333333, "file format"=enum."binary", "power(V)"=2.1, "Magn Field(T) "=0.0}, {"temperature"=50.759, "temperature str"="50.75900", "file path"=path "D:/Data/Ultrasound/LSCO/LSCO22__130814c/5_Cooling_2nd_try/September_2014/091714/50.75900K_500_2500_2.10000V_0.00000T_Sep17-2014__11-41-42_001_091714.bin", "last mod"=timestamp(3493813302 s since 1904-01-01), "file name str"="D:\\Data\\Ultrasound\\LSCO\\LSCO22__130814c\\5_Cooling_2nd_try\\September_2014\\091714\\50.75900K_500_2500_2.10000V_0.00000T_Sep17-2014__11-41-42_001_091714.bin", "mod time(min)"=58230221.7, "file format"=enum."binary", "power(V)"=2.1, "Magn Field(T) "=0.0}, {"temperature"=50.695, "temperature str"="50.69500", "file path"=path "D:/Data/Ultrasound/LSCO/LSCO22__130814c/5_Cooling_2nd_try/September_2014/091714/50.69500K_500_2500_2.10000V_0.00000T_Sep17-2014__11-43-01_001_091714.bin", "last mod"=timestamp(3493813381 s since 1904-01-01), "file name str"="D:\\Data\\Ultrasound\\LSCO\\LSCO22__130814c\\5_Cooling_2nd_try\\September_2014\\091714\\50.69500K_500_2500_2.10000V_0.00000T_Sep17-2014__11-43-01_001_091714.bin", "mod time(min)"=58230223.016666666, "file format"=enum."binary", "power(V)"=2.1, "Magn Field(T) "=0.0}, {"temperature"=50.631, "temperature str"="50.63100", "file path"=path "D:/Data/Ultrasound/LSCO/LSCO22__130814c/5_Cooling_2nd_try/September_2014/091714/50.63100K_500_2500_2.10000V_0.00000T_Sep17-2014__11-44-21_001_091714.bin", "last mod"=timestamp(3493813461 s since 1904-01-01), "file name str"="D:\\Data\\Ultrasound\\LSCO\\LSCO22__130814c\\5_Cooling_2nd_try\\September_2014\\091714\\50.63100K_500_2500_2.10000V_0.00000T_Sep17-2014__11-44-21_001_091714.bin", "mod time(min)"=58230224.35, "file format"=enum."binary", "power(V)"=2.1, "Magn Field(T) "=0.0}, {"temperature"=50.566, "temperature str"="50.56600", "file path"=path "D:/Data/Ultrasound/LSCO/LSCO22__130814c/5_Cooling_2nd_try/September_2014/091714/50.56600K_500_2500_2.10000V_0.00000T_Sep17-2014__11-45-40_001_091714.bin", "last mod"=timestamp(3493813540 s since 1904-01-01), "file name str"="D:\\Data\\Ultrasound\\LSCO\\LSCO22__130814c\\5_Cooling_2nd_try\\September_2014\\091714\\50.56600K_500_2500_2.10000V_0.00000T_Sep17-2014__11-45-40_001_091714.bin", "mod time(min)"=58230225.666666664, "file format"=enum."binary", "power(V)"=2.1, "Magn Field(T) "=0.0}, {"temperature"=50.499, "temperature str"="50.49900", "file path"=path "D:/Data/Ultrasound/LSCO/LSCO22__130814c/5_Cooling_2nd_try/September_2014/091714/50.49900K_500_2500_2.10000V_0.00000T_Sep17-2014__11-46-59_001_091714.bin", "last mod"=timestamp(3493813619 s since 1904-01-01), "file name str"="D:\\Data\\Ultrasound\\LSCO\\LSCO22__130814c\\5_Cooling_2nd_try\\September_2014\\091714\\50.49900K_500_2500_2.10000V_0.00000T_Sep17-2014__11-46-59_001_091714.bin", "mod time(min)"=58230226.983333334, "file format"=enum."binary", "power(V)"=2.1, "Magn Field(T) "=0.0}, {"temperature"=50.428, "temperature str"="50.42800", "file path"=path "D:/Data/Ultrasound/LSCO/LSCO22__130814c/5_Cooling_2nd_try/September_2014/091714/50.42800K_500_2500_2.10000V_0.00000T_Sep17-2014__11-48-19_001_091714.bin", "last mod"=timestamp(3493813699 s since 1904-01-01), "file name str"="D:\\Data\\Ultrasound\\LSCO\\LSCO22__130814c\\5_Cooling_2nd_try\\September_2014\\091714\\50.42800K_500_2500_2.10000V_0.00000T_Sep17-2014__11-48-19_001_091714.bin", "mod time(min)"=58230228.31666667, "file format"=enum."binary", "power(V)"=2.1, "Magn Field(T) "=0.0}, {"temperature"=50.361, "temperature str"="50.36100", "file path"=path "D:/Data/Ultrasound/LSCO/LSCO22__130814c/5_Cooling_2nd_try/September_2014/091714/50.36100K_500_2500_2.10000V_0.00000T_Sep17-2014__11-49-38_001_091714.bin", "last mod"=timestamp(3493813778 s since 1904-01-01), "file name str"="D:\\Data\\Ultrasound\\LSCO\\LSCO22__130814c\\5_Cooling_2nd_try\\September_2014\\091714\\50.36100K_500_2500_2.10000V_0.00000T_Sep17-2014__11-49-38_001_091714.bin", "mod time(min)"=58230229.63333333, "file format"=enum."binary", "power(V)"=2.1, "Magn Field(T) "=0.0}, {"temperature"=50.295, "temperature str"="50.29500", "file path"=path "D:/Data/Ultrasound/LSCO/LSCO22__130814c/5_Cooling_2nd_try/September_2014/091714/50.29500K_500_2500_2.10000V_0.00000T_Sep17-2014__11-50-58_001_091714.bin", "last mod"=timestamp(3493813858 s since 1904-01-01), "file name str"="D:\\Data\\Ultrasound\\LSCO\\LSCO22__130814c\\5_Cooling_2nd_try\\September_2014\\091714\\50.29500K_500_2500_2.10000V_0.00000T_Sep17-2014__11-50-58_001_091714.bin", "mod time(min)"=58230230.96666667, "file format"=enum."binary", "power(V)"=2.1, "Magn Field(T) "=0.0}, {"temperature"=50.232, "temperature str"="50.23200", "file path"=path "D:/Data/Ultrasound/LSCO/LSCO22__130814c/5_Cooling_2nd_try/September_2014/091714/50.23200K_500_2500_2.10000V_0.00000T_Sep17-2014__11-52-17_001_091714.bin", "last mod"=timestamp(3493813937 s since 1904-01-01), "file name str"="D:\\Data\\Ultrasound\\LSCO\\LSCO22__130814c\\5_Cooling_2nd_try\\September_2014\\091714\\50.23200K_500_2500_2.10000V_0.00000T_Sep17-2014__11-52-17_001_091714.bin", "mod time(min)"=58230232.28333333, "file format"=enum."binary", "power(V)"=2.1, "Magn Field(T) "=0.0}, {"temperature"=50.162, "temperature str"="50.16200"
